vi "PM100D_Plot_ph.vi"(1 "Meas Time (s)":dbl=nan, 2 "Beam Name":string="Green Unshifted") -> (0 "Array":dbl[](array[numeric]))   [LabVIEW 2015]
doc: "This VI shows how to communicate with a PM100D optical power/energy meter with SCPI commands.\n- Initializing the instrument\n- Getting system info\n- Setting parameters\n- Measurement configuration\n- Measuring queue\n- Fetching and displaying a measurement value\n- Closing the application"
panel:
  in  "Publish As Adam Channel":bool
  out "Wavelength nm":string="488"
  out "Waveform Chart":dbl(graph)
  out "Readout value":dbl format="%^#_9e"
  out "IDN String":string
  out "Sensor SN":string
  out "Sensor Name":string
  out "Sensor Flags":bool[](array[boolean])
  out "New":bool
  in  "Timeout [ms]":i32=1000
  in  "stop":bool
  in  "Readout Config":string(combo)="POW"
  out "Readout string":string
  out "Error log":string
  in  "Averaging Rate":i32=300
  # "1 Power Sensor"
  # "2 Energy Sensor"
  # "4"
  # "8"
  # "16 Response settable"
  # "32 Wavelength settable"
  # "64 Tau (time constant) settable"
  # "128"
  # "256 With temperature sensor"
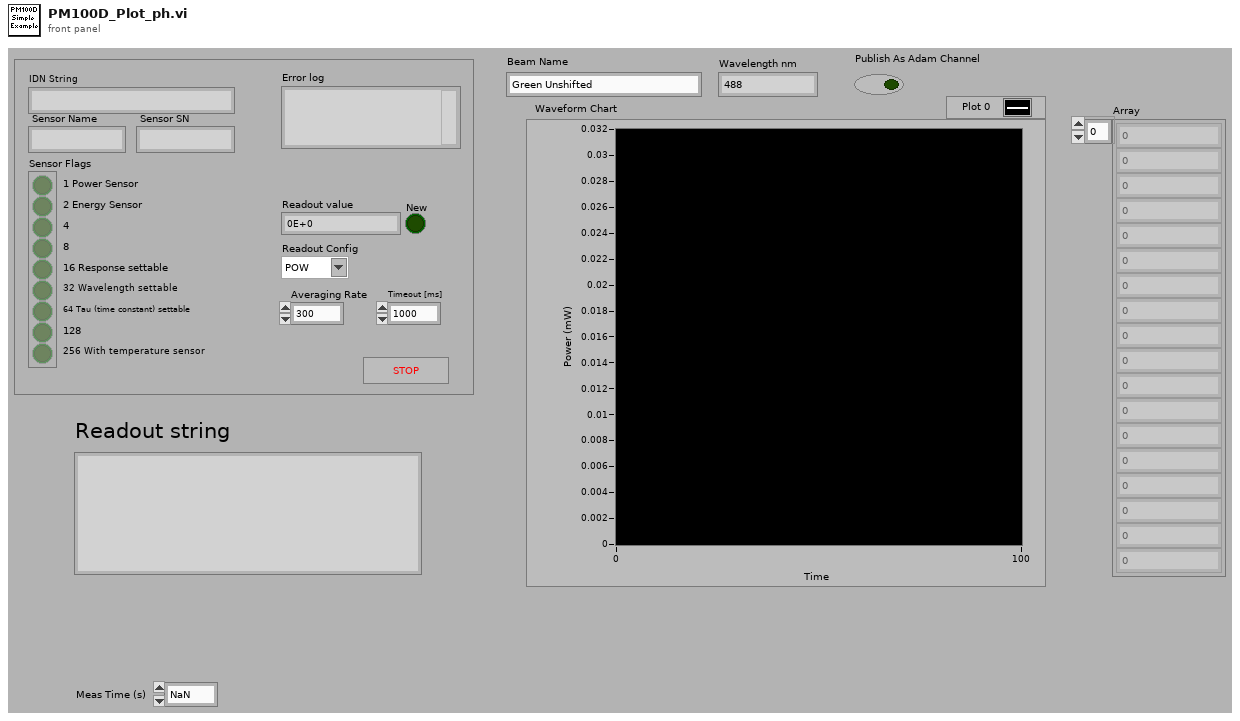
[diagram p1: front panel]
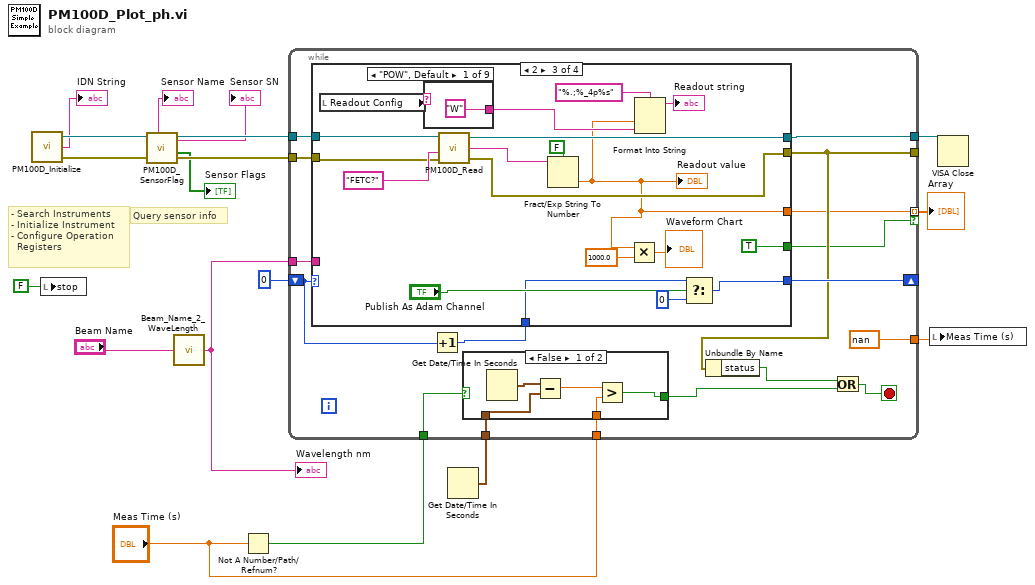
[diagram p0: block diagram]
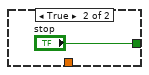
[diagram p2: hidden frame]
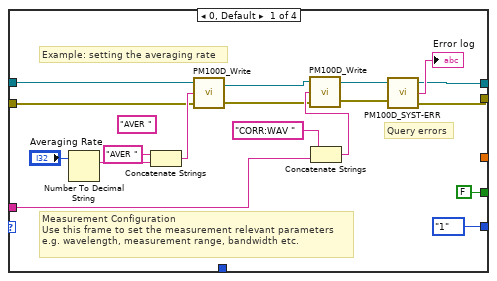
[diagram p3: hidden frame]
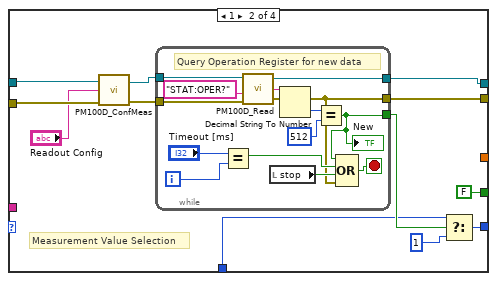
[diagram p4: hidden frame]
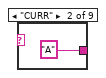
[diagram p5: hidden frame]
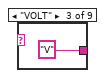
[diagram p6: hidden frame]
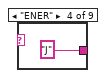
[diagram p7: hidden frame]
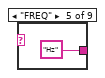
[diagram p8: hidden frame]
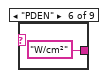
[diagram p9: hidden frame]
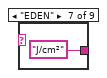
[diagram p10: hidden frame]
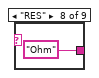
[diagram p11: hidden frame]
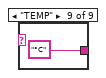
[diagram p12: hidden frame]
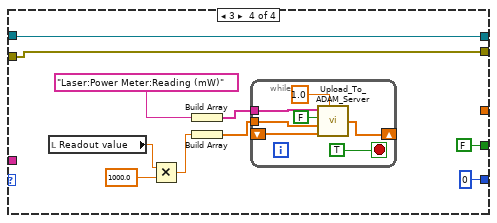
[diagram p13: hidden frame]
diagram:
  # "- Search Instruments\n- Initialize Instrument\n- Configure Operation\n  Registers"
  # "Query sensor info"
  n1 = call "PM100D_Initialize.vi"() -> ("error out"=w17:errorcluster, "Instrument"=→"IDN String":string, "VISA out"=w18:refnum<visa-resource-name>)  [unwired: 3 out]
  n2 = local write "stop"(FALSE ("stop")) -> ()
  n3 = call "PM100D_SensorFlag.vi"("error in (no error)"=w17, "VISA in"=w18) -> ("error out"=w15:errorcluster, "flags"=→"Sensor Flags":bool[], "VISA out"=w16:refnum<visa-resource-name>, "sn"=→"Sensor SN":string, "name"=→"Sensor Name":string)  [unwired: 5 out]
  n4 = call "Beam_Name_2_WaveLength.vi"("Beam Name"="Beam Name") -> ("Wavelength nm"=w8:string)
  "Wavelength nm" <- w8
  n5 = Not A Number/Path/Refnum?(number/path/refnum="Meas Time (s)") -> (NaN/Path/Refnum?=w4:bool)
  n6 = Get Date/Time In Seconds() -> (seconds since 1Jan1904=w3:timestamp)
  n7 = while {
    tunnel: w16 -> [w35]
    tunnel: w15 -> [w34]
    shift-right: [w33] -> _
    shift-left: 0 -> [w30]
    tunnel: [w32] -> w6
    tunnel: [w27] -> _
    tunnel: w8 -> [w31]
    tunnel: [w25] -> w5 mode=indexing if=w24
    tunnel: w4 -> [w23]
    tunnel: w3 -> [w21]
    tunnel: "Meas Time (s)" -> [w20]
    tunnel: [nan ("Meas Time (s)")] -> w1
    stop <- w28 stop-if-true
    n8 = Increment(x=w30) -> (x+1=w29:i32)
    n9 = case shown="2" w30 {
      tunnel: w35 -> [w56 w71 w103 w123]
      tunnel: w34 -> [w53 w70 w102 w122]
      tunnel: [enum16{"0", "1", "2"}."1" w65 w92 0 ("f")] -> w33
      tunnel: [w51 w67 w101 w123] -> w32
      tunnel: [w50 w66 w94 w122] -> w27
      tunnel: w31 -> [w47 _ _ _]
      tunnel: w29 -> [_ w62 w91 _]
      tunnel: [_ _ w88 _] -> w25
      tunnel: [FALSE FALSE TRUE FALSE] -> w24
      frame 0, Default {
        (unwired) "AVER " ("string")
        # "Query errors"
        # "Example: setting the averaging rate"
        # "Measurement Configuration\nUse this frame to set the measurement relevant parameters\ne.g. wavelength, measurement range, bandwidth etc."
        n10 = Number To Decimal String(number="Averaging Rate") -> (decimal integer string=w58:string)  [unwired: 1 out]
        n11 = Concatenate Strings("AVER " ("string"), w58) -> (w55:string)
        n12 = call "PM100D_Write.vi"("error in (no error)"=w53, "Command"=w55, "VISA in"=w56) -> ("error out"=w45:errorcluster, "VISA out"=w46:refnum<visa-resource-name>)
        n13 = Concatenate Strings("CORR:WAV " ("string"), w47) -> (w49:string)
        n14 = call "PM100D_Write.vi"("error in (no error)"=w45, "Command"=w49, "VISA in"=w46) -> ("error out"=w44:errorcluster, "VISA out"=w43:refnum<visa-resource-name>)
        n15 = call "PM100D_SYST-ERR.vi"("error out 2"=w44, "VISA In"=w43) -> ("error out"=w50:errorcluster, "Error"=→"Error log":string, "VISA Out"=w51:refnum<visa-resource-name>)  [unwired: 1 out]
      }
      frame 1 {
        # "Measurement Value Selection"
        n16 = call "PM100D_ConfMeas.vi"("error in"=w70, "Conf:"="Readout Config", "VISA In"=w71) -> ("error out"=w68:errorcluster, "dup VISA session"=w69:refnum<visa-resource-name>)
        n17 = while {
          tunnel: w69 -> [w81]
          tunnel: w68 -> [w80]
          tunnel: [w79] -> w67
          tunnel: [w72] -> w66
          tunnel: [w73] -> w64
          i -> [w75]
          stop <- w77 stop-if-true
          # "Query Operation Register for new data"
          n18 = Equal?(x="Timeout [ms]", y=w75) -> (x = y?=w74:bool)
          n19 = call "PM100D_Read.vi"("error in (no error)"=w80, "Command"="STAT:OPER?", "VISA in"=w81) -> ("error out"=w72:errorcluster, "ReadValue"=w84:string, "VISA out"=w79:refnum<visa-resource-name>)  [unwired: 1 out]
          n20 = local read "stop"() -> (w78:bool)
          n21 = Decimal String To Number(string=w84) -> (number=w83:i32)  [unwired: 2 in, 1 out]
          n22 = Equal?(x=w83, y=512) -> (x = y?=w73:bool)
          "New" <- w73
          n23 = Compound Arithmetic op=OR(w73, w74, w78, w72) -> (w77:bool)
        }
        n24 = Select(t=w62, s=w64, f=1) -> (s? t:f=w65:i32)
      }
      frame 2 {
        n25 = local read "Readout Config"() -> (w100:string)
        n26 = case shown="\"POW\", Default" w100 {
          tunnel: ["W" "A" "V" "J" "Hz" "W/cm²" "J/cm²" "Ohm" "°C"] -> w96
          frame "POW", Default {
          }
          frame "CURR" {
          }
          frame "VOLT" {
          }
          frame "ENER" {
          }
          frame "FREQ" {
          }
          frame "PDEN" {
          }
          frame "EDEN" {
          }
          frame "RES" {
          }
          frame "TEMP" {
          }
        }
        n27 = call "PM100D_Read.vi"("error in (no error)"=w102, "Command"="FETC?", "VISA in"=w103) -> ("error out"=w94:errorcluster, "ReadValue"=w99:string, "VISA out"=w101:refnum<visa-resource-name>)  [unwired: 1 out]
        n28 = Fract/Exp String To Number(use system decimal point (T)=FALSE, string=w99) -> (number=w88:dbl)  [unwired: 3 out]
        "Readout value" <- w88
        n29 = Multiply(x=w88, y=1000.0) -> (x*y=→"Waveform Chart":dbl)
        n30 = Format Into String(format string="%.;%_4p%s", w88, w96) -> (resulting string=→"Readout string":string)  [unwired: 2 in, 1 out]
        n31 = Select(t=w91, s="Publish As Adam Channel", f=0) -> (s? t:f=w92:i32)
      }
      frame 3 {
        n32 = local read "Readout value"() -> (w117:dbl)
        n33 = Multiply(x=w117, y=1000.0) -> (x*y=w115:dbl)
        n34 = Build Array("Laser:Power Meter:Reading (mW)" ("String")) -> (w118:string[])
        n35 = Build Array(w115) -> (w119:dbl[])
        n36 = while {
          shift-right: [w130] -> _
          shift-left: _ -> [w129]
          tunnel: w119 -> [w126]
          tunnel: w118 -> [w125]
          stop <- TRUE stop-if-true
          n37 = call "Upload_To_ADAM_Server.vi"("Averaging Period (s)"=1.0, "Shift In"=w129, "Channel Values"=w126, "Give Variance"=FALSE, "Channel Names"=w125) -> ("Shift Out"=w130:dbl[])  [unwired: 1 in]
        }
      }
    }
    n38 = case shown="False" w23 {
      tunnel: [w36 "stop"] -> w22
      tunnel: w21 -> [w39 _]
      tunnel: w20 -> [w37 _]
      frame False {
        n39 = Get Date/Time In Seconds() -> (seconds since 1Jan1904=w40:timestamp)
        n40 = Subtract(x=w40, y=w39) -> (x-y=w38:dbl)
        n41 = Greater?(x=w38, y=w37) -> (0:w36:bool)
      }
      frame True {
      }
    }
    n42 = Unbundle By Name(w27) -> ("status"=w26:bool)
    n43 = Or(x=w26, y=w22) -> (x .or. y?=w28:bool)
  }
  "Array" <- w5
  n44 = local write "Meas Time (s)"(w1) -> ()
  n45 = VISA Close(VISA resource name=w6) -> ()  [unwired: 1 in, 1 out]
